vi "DSF Version.vi"() -> (0 "dsf version":T1)   [LabVIEW 2021, in "DSF Core.lvlib"]
uses:
  DSF Core.lvlib
  Typedefs/DSF Version Info.ctl
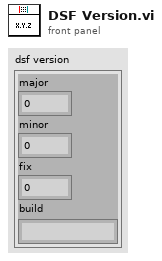
[diagram p1: front panel]
types:
  T1 = typedef "DSF Core.lvlib/DSF Version Info.ctl" = cluster{"major":u32, "minor":u32, "fix":u32, "build":string}
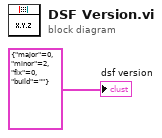
[diagram p0: block diagram]
diagram:
  "dsf version" <- T1 {"major"=0, "minor"=2, "fix"=0, "build"=""} ("dsf version")
